vi "Command Handler.vi"(8 "error in (no error)":errorcluster, 11 "J1939 Main Configuration":T1={"Parameters"={"J1939 XNET Settings"={"XNET Database"="", "XNET Cluster"="", "CAN Port"="", "Baud rate [Bd]"=0, "Termination"=0, "Incoming Rate"=0, "Outcoming Rate"=1, "Write Decimation"=1}, "Incoming Single Point Configuraiton"={"ID"=[], "Conversion"=[], "Channel Array Positions"=[], "Frame Length"=[]}, "Outgoing Cyclic Configuraiton"={"ID"=[], "Conversion"=[], "Channel Array Positions"=[], "Frame Length"=[], "Transmit Propreties"=[]}, "J1939 Monitor Settings"={"J1939 Network Address"=0, "Name"=0}, "Simulated Addresses"=[], "Simulated Addresses LUT"=variant, "Name"=""}, "Name"="", "J1939 Cluster"={"Processed Incoming"=refnum, "Current Device Address"=0, "Processed Outgoing"=refnum, "Process Outgoing"=refnum, "Name"=0}, "References"={"BAM Buffer"=refnum, "CM Buffer"=refnum, "CM Gen"=refnum, "BAM Gen"=refnum, "Address Claims"=refnum, "RQST"=refnum}, "Frame In"="", "Frame Out"="", "Incoming Timeout"=0, "Outgoing Timeout"=0, "Process"=refnum, "Data Ref"=refnum, "Scale Ref"=refnum, "Incoming Direct Access"={"Offset"=0, "Length"=0}, "Outgoing Direct Access"={"Offset"=0, "Length"=0}, "Name and Address"="", "Simulated Addresses"=[], "Simulated Addresses LUT"=variant, "Outgoing"=refnum, "Incoming"=refnum, "Comm"=refnum} {"Simulated Addresses"."Simulated Addresses"."J1939 XNET Settings"."Name" format="%.0x"; "Simulated Addresses"."Simulated Addresses"."DM1 Data"."Data Reference" format="%.0x"; "Simulated Addresses"."Simulated Addresses"."DM1 Enable?"."Data Reference" format="%.0x"; "Simulated Addresses"."Simulated Addresses"."DM2 Data"."Data Reference" format="%.0x"; "Simulated Addresses"."Simulated Addresses"."DM2 Enable?"."Data Reference" format="%.0x"; "Parameters"."Simulated Addresses"."Simulated Addresses"."J1939 XNET Settings"."Name" format="%.0x"; "Parameters"."J1939 Monitor Settings"."Name" format="%.0x"; "Parameters"."Outgoing Cyclic Configuraiton"."Transmit Propreties"."Transmit Time" format="%#_p"; "Parameters"."J1939 XNET Settings"."Termination" items=["Off", "On"]}) -> (0 "error out":errorcluster)   [LabVIEW 2015, in "J1939 Addon Engine.lvlib"]
uses:
  J1939 Addon Engine.lvlib
  Types/Configuration Cluster.ctl
  <vilib>/NI/NIVS Inline Async API/_VS Inline Async API/Process/Process.lvclass
  <vilib>/NI/NIVS Addon Network Comm/Engine/VeriStand Comm.lvclass
  Types/Process Parameters.ctl
  Shared/Types/XNET Settings.ctl
  Types/Incoming Single Point Configuration.ctl
  Types/Outgoing Cyclic Configuration.ctl
  Shared/Types/XNET Frame Event Properties.ctl
  Shared/Types/Monitor Settings.ctl
  Types/Simulated Settings.ctl
  Shared/Types/Compiled Simulated Settings.ctl
  <vilib>/NI Veristand/Custom Device API/Block Data Reference.ctl
  <vilib>/NI Veristand/Custom Device API/Data Reference.ctl
  Types/DTC FIFOs.ctl
  J1939 Multi Packet Frame/Types/Setup Information Cluster.ctl
  <vilib>/xnet/xnet.llb/XNET Frame CAN.ctl
  <vilib>/xnet/xnet.llb/XNET Frame Type CAN.ctl
  Shared/J1939 Utilities/Types/CAN Outgoing Message Cluster.ctl
  J1939 Multi Packet Frame/Types/TP List References.ctl
  J1939 Multi Packet Frame/Types/BAM Buffer Connections List_Ref.ctl
  J1939 Multi Packet Frame/Types/TP Buffer Connection Cluster.ctl
  J1939 Multi Packet Frame/Types/Connection Mode Generation Connection Ref.ctl
  J1939 Multi Packet Frame/Types/Connection Mode Generation Connection Cluster.ctl
  J1939 Multi Packet Frame/Types/BAM Generation Connections List_Ref.ctl
  J1939 Multi Packet Frame/Types/BAM Generation Connection Cluster.ctl
  J1939 Multi Packet Frame/Types/Address Table Reference.ctl
  J1939 Multi Packet Frame/Types/RQST Lookup Table Reference.ctl
  Types/Data Lookup Table Reference.ctl
  Types/Datatable Lookup DVR.ctl
  Types/Conversion Lookup Table Reference.ctl
  <vilib>/NI/NIVS Inline Async API/_Data Access Engine/Access Type Classes/Read/Read.lvclass
  <vilib>/NI/NIVS Inline Async API/_Data Access Engine/Access Type Classes/Write/Write.lvclass
  <vilib>/NI/NIVS Addon Network Comm/Engine/VeriStand Comm.lvclass/VeriStand Comm.ctl
  Shared/Types/Request Message.ctl
  J1939 Multi Packet Frame/Types/Address Lookup Table Action.ctl
  <vilib>/NI/NIVS Inline Async API/_VS Inline Async API/Process/Process.lvclass/Process.ctl
  <vilib>/NI/NIVS Inline Async API/_VS Inline Async API/Error Handling Process/SubVIs/Error.ConvertArray.vi
  <vilib>/NI/AMC/Read Next Message.vi
  <vilib>/NI/Tools/Keyed Array/Index.vi
  Shared/J1939 Utilities/Common Messages.vi
  Shared/J1939 Utilities/SubVIs/Request.vi
  J1939 Multi Packet Frame/SubVIs/RQST Lookup Table Act.vi
  <vilib>/NI/AMC/Send Local Message.vi
  <vilib>/NI/AMC/Read Termination Message.vi
  <vilib>/NI/Tools/Keyed Array/Map String.vi
  Shared/J1939 Utilities/Common Conversions.vi
  Shared/J1939 Utilities/SubVIs/Convert J1939 ID to CAN Arb ID.vi
  <vilib>/NI/AMC/Create Single Message.vi
  <vilib>/NI/AMC/Update Message Routing Info.vi
  <vilib>/NI/Tools/String/Get Case Matching.vi
  <vilib>/NI/AMC/Send Message.vi
  J1939 Multi Packet Frame/SubVIs/Address Lookup Table.vi
  <vilib>/xnet/xnet.llb/XNET Read (State CAN Comm).vi
  J1939 Multi Packet Frame/SubVIs/RQST Lookup Table.vi
  <vilib>/NI/AMC/Globals.vi
  <vilib>/NI/NIVS Addon Network Comm/Shared/Comm Constants.vi
  Shared/J1939 Addon Shared.lvlib
  Shared/J1939 Utilities/J1939 Utilities.lvlib
  <vilib>/NI Veristand/Custom Device Tools/Custom Device Utility Library/Custom Device Utility Library.lvlib
  <vilib>/NI VeriStand/Custom Device API/Custom Device API.lvlib
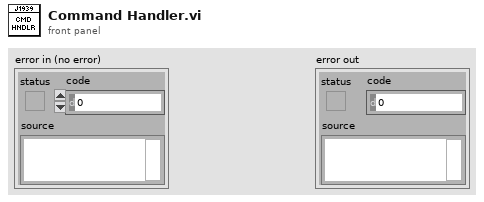
[diagram p1: front panel]
types:
  T1 = typedef "J1939 Addon Engine.lvlib/Configuration Cluster.ctl" = cluster{"Parameters":T2, "Name":string, "J1939 Cluster":T13, "References":T14, "Frame In":refnum<k21>, "Frame Out":refnum<k21>, "Incoming Timeout":u32, "Outgoing Timeout":u32, "Process":refnum<class "Process.lvclass">, "Data Ref":T20, "Scale Ref":T21, "Incoming Direct Access":cluster{"Offset":u32, "Length":u32}, "Outgoing Direct Access":cluster{"Offset":u32, "Length":u32}, "Name and Address":string, "Simulated Addresses":T8[], "Simulated Addresses LUT":variant, "Outgoing":refnum<data-value>, "Incoming":refnum<data-value>, "Comm":refnum<class "VeriStand Comm.lvclass">}
  T2 = typedef "J1939 Addon Engine.lvlib/Process Parameters.ctl" = cluster{"J1939 XNET Settings":T3, "Incoming Single Point Configuraiton":T4, "Outgoing Cyclic Configuraiton":T5, "J1939 Monitor Settings":T7, "Simulated Addresses":T8[], "Simulated Addresses LUT":variant, "Name":string}
  T3 = typedef "J1939 Addon Shared.lvlib/XNET Settings.ctl" = cluster{"XNET Database":refnum<k21>, "XNET Cluster":refnum<k21>, "CAN Port":string, "Baud rate [Bd]":u32, "Termination":u32, "Incoming Rate":u32, "Outcoming Rate":u32, "Write Decimation":u32}
  T4 = typedef "J1939 Addon Engine.lvlib/Incoming Single Point Configuration.ctl" = cluster{"ID":u32[], "Conversion":refnum<k21>[], "Channel Array Positions":cluster{"Offset":u32, "Length":u32}[], "Frame Length":u32[]}
  T5 = typedef "J1939 Addon Engine.lvlib/Outgoing Cyclic Configuration.ctl" = cluster{"ID":u32[], "Conversion":refnum<k21>[], "Channel Array Positions":cluster{"Offset":u32, "Length":u32}[], "Frame Length":u32[], "Transmit Propreties":T6[]}
  T6 = typedef "J1939 Addon Shared.lvlib/XNET Frame Event Properties.ctl" = cluster{"Transmit trigger":enum16{"Channel value change"}, "Enable software cyclic trigger":bool, "Transmit Time":dbl}
  T7 = typedef "J1939 Addon Shared.lvlib/Monitor Settings.ctl" = cluster{"J1939 Network Address":u8, "Name":u64}
  T8 = typedef "J1939 Addon Engine.lvlib/Simulated Settings.ctl" = cluster{"Simulated Addresses":T9, "FIFOs":T12}
  T9 = typedef "J1939 Addon Shared.lvlib/Compiled Simulated Settings.ctl" = cluster{"J1939 XNET Settings":T7, "DM1 Data":T10[], "DM1 Data":dbl[], "DM1 Enable?":T10[], "DM1 Enable?":dbl[], "DM2 Data":T10[], "DM2 Data":dbl[], "DM2 Enable?":T10[], "DM2 Enable?":dbl[]}
  T10 = typedef "Custom Device API.lvlib/Block Data Reference.ctl" = cluster{"Data Reference":T11, "Offset":u64, "Length":u64}
  T11 = typedef "Custom Device API.lvlib/Data Reference.ctl" = i32
  T12 = typedef "J1939 Addon Engine.lvlib/DTC FIFOs.ctl" = cluster{"DM1 Data":refnum<k33>, "DM1 Enable?":refnum<k33>, "DM2 Data":refnum<k33>, "DM2 Enable?":refnum<k33>, "DM1 Reset?":refnum<k33>, "DM2 Reset?":refnum<k33>}
  T13 = typedef "J1939 Addon Engine.lvlib/Setup Information Cluster.ctl" = cluster{"Processed Incoming":refnum<queue>, "Current Device Address":u8, "Processed Outgoing":refnum<queue>, "Process Outgoing":refnum<queue>, "Name":u64}
  T14 = typedef "J1939 Addon Engine.lvlib/TP List References.ctl" = cluster{"BAM Buffer":T15, "CM Buffer":T15, "CM Gen":T16, "BAM Gen":T17, "Address Claims":T18, "RQST":T19}
  T15 = typedef "J1939 Addon Engine.lvlib/BAM Buffer Connections List_Ref.ctl" = refnum<data-value>
  T16 = typedef "J1939 Addon Engine.lvlib/Connection Mode Generation Connection Ref.ctl" = refnum<data-value>
  T17 = typedef "J1939 Addon Engine.lvlib/BAM Generation Connections List_Ref.ctl" = refnum<data-value>
  T18 = typedef "J1939 Addon Engine.lvlib/Address Table Reference.ctl" = refnum<data-value>
  T19 = typedef "J1939 Addon Engine.lvlib/RQST Lookup Table Reference.ctl" = refnum<data-value>
  T20 = typedef "J1939 Addon Engine.lvlib/Data Lookup Table Reference.ctl" = refnum<data-value>
  T21 = typedef "J1939 Addon Engine.lvlib/Conversion Lookup Table Reference.ctl" = refnum<data-value>
  T22 = typedef "J1939 Addon Shared.lvlib/Request Message.ctl" = cluster{"PGN":u32, "DA":u8, "Ignore Response":bool}
  T23 = typedef "J1939 Addon Shared.lvlib/J1939 Utilities.lvlib/CAN Outgoing Message Cluster.ctl" = cluster{"Identifier":u32, "Data":u8[]}
  T24 = typedef "J1939 Addon Engine.lvlib/Address Lookup Table Action.ctl" = enum16{"Initialize", "Add", "Get", "Remove", "Get All"}
  T25 = typedef "NI VeriStand Addon Network Comm.lvlib/VeriStand Comm.lvclass/Response Information.ctl" = cluster{"response name":string, "responseQ":string}
  T26 = typedef "XNET Frame CAN.ctl" = cluster{"timestamp":timestamp, "payload":u8[], "identifier":u32, "type":T27, "extended?":bool, "echo?":bool}
  T27 = typedef "XNET Frame Type CAN.ctl" = u8
  T28 = typedef "XNET CAN Comm.ctl" = cluster{"fault code":i32, "fault?":bool, "communication state":T29, "last error":T30, "receive error counter":u8, "transmit error counter":u8, "transceiver error?":bool, "sleep?":bool}
  T29 = typedef "XNET CAN Comm State.ctl" = u8
  T30 = typedef "XNET CAN Last Err.ctl" = u8
  T31 = typedef "J1939 Addon Shared.lvlib/Address Lookup Table Data.ctl" = cluster{"Name":u8[], "Address":u8}
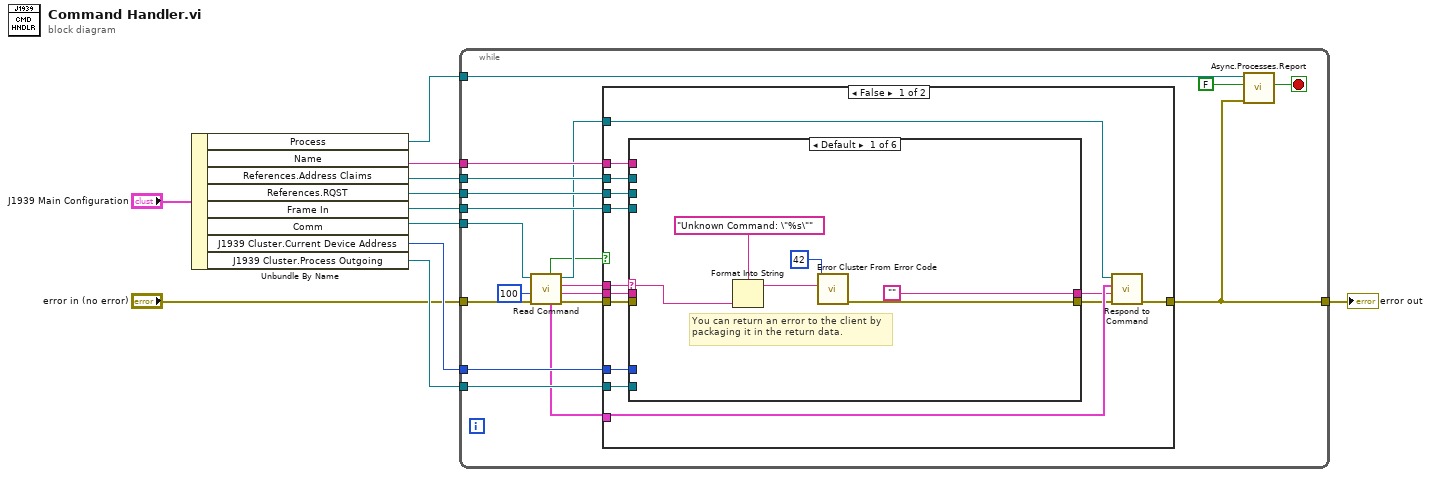
[diagram p0: block diagram]
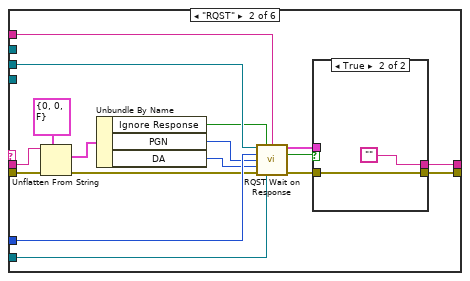
[diagram p2: hidden frame]
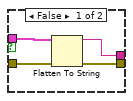
[diagram p3: hidden frame]
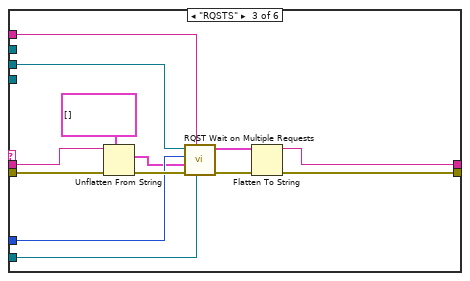
[diagram p4: hidden frame]
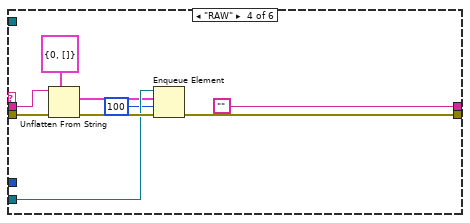
[diagram p5: hidden frame]
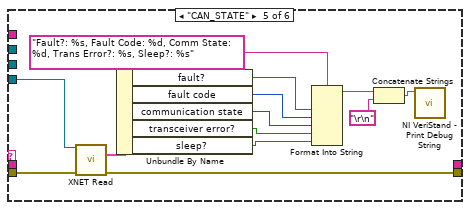
[diagram p6: hidden frame]
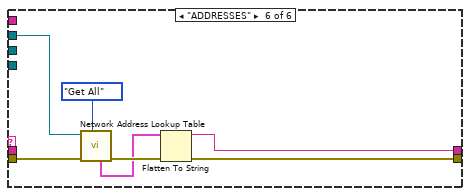
[diagram p7: hidden frame]
diagram:
  n1 = Unbundle By Name("J1939 Main Configuration") -> ("Process"=w11:refnum<class "Process.lvclass">, "Name"=w10:string, "References.Address Claims"=w9:T18, "References.RQST"=w8:T19, "Frame In"=w7:refnum<k21>, "Comm"=w6:refnum<class "VeriStand Comm.lvclass">, "J1939 Cluster.Current Device Address"=w5:u8, "J1939 Cluster.Process Outgoing"=w4:refnum<queue>)
  n2 = while {
    tunnel: "error in (no error)" -> [w27]
    tunnel: [w19] -> w1
    tunnel: w11 -> [w29]
    tunnel: w6 -> [w26]
    tunnel: w10 -> [w25]
    tunnel: w7 -> [w24]
    tunnel: w4 -> [w23]
    tunnel: w5 -> [w22]
    tunnel: w8 -> [w21]
    tunnel: w9 -> [w20]
    stop <- w30 stop-if-true
    n3 = call <vilib>:"Read Command.vi"("error in (no error)"=w27, "timeout (100 ms)"=100, "VeriStand Comm in"=w26) -> ("error out"=w17:errorcluster, "message value"=w15:string, "message name"=w16:string, "VeriStand Comm out"=w13:refnum<class "VeriStand Comm.lvclass">, "ResponseInfo"=w14:T25, "timed out?"=w12:bool)  [unwired: 3 in]
    n4 = case shown="False" w12 {
      tunnel: w25 -> [w44 _]
      tunnel: w24 -> [w43 _]
      tunnel: w23 -> [w42 _]
      tunnel: w22 -> [w41 _]
      tunnel: w21 -> [w40 _]
      tunnel: w20 -> [w39 _]
      tunnel: [w38 w116] -> w19
      tunnel: w17 -> [w37 w116]
      tunnel: w16 -> [w36 _]
      tunnel: w15 -> [w35 _]
      tunnel: w14 -> [w34 _]
      tunnel: w13 -> [w33 _]
      frame False {
        n5 = case shown="Default" w36 {
          selector: w36 -> [w46 _ _ _ _ _]
          tunnel: w35 -> [_ w54 w83 w94 _ _]
          tunnel: [w47 w66 w86 w88 w106 w109] -> w31
          tunnel: ["" ("data string") w63 w85 "" _ w110] -> w32
          tunnel: w42 -> [_ w61 w80 w91 _ _]
          tunnel: w37 -> [_ w60 w84 w95 w108 w114]
          tunnel: w40 -> [_ w53 w78 _ _ _]
          tunnel: w41 -> [_ w67 w77 _ _ _]
          tunnel: w39 -> [_ _ _ _ _ w113]
          tunnel: w44 -> [_ w51 w74 _ _ _]
          tunnel: w43 -> [_ _ _ _ w107 _]
          frame Default {
            # "You can return an error to the client by packaging it in the return data."
            n6 = Format Into String(format string="Unknown Command: \"%s\"", w46) -> (resulting string=w48:string)  [unwired: 2 in, 1 out]
            n7 = call <vilib>:"Error Cluster From Error Code.vi"("error message (\"\")"=w48, "error code (0)"=42) -> ("error out"=w47:errorcluster)  [unwired: 7 in]
          }
          frame "RQST" {
            n8 = Unflatten From String(type=T22 {"PGN"=0, "DA"=0, "Ignore Response"=FALSE} ("Cluster"), binary string=w54, error in (no error)=w60) -> (value=w57:T22, error out=w59:errorcluster)  [unwired: 2 in, 1 out]
            n9 = Unbundle By Name(w57) -> ("Ignore Response"=w52:bool, "PGN"=w56:u32, "DA"=w55:u8)
            n10 = call "RQST Wait on Response.vi"("ref in"=w53, "Ignore Response"=w52, "Name"=w51, "Source Address"=w67, "PGN"=w56, "DA"=w55, "error in (no error)"=w59, "Processed Outgoing"=w61) -> ("element"=w62:T26, "timed out?"=w64:bool, "error out"=w65:errorcluster)  [unwired: 4 in, 1 out]
            n11 = case shown="True" w64 {
              tunnel: [w69 w73] -> w66
              tunnel: w65 -> [w70 w73]
              tunnel: [w68 ""] -> w63
              tunnel: w62 -> [w71 _]
              frame False {
                n12 = Flatten To String(anything=w71, error in (no error)=w70) -> (data string=w68:string, error out=w69:errorcluster)  [unwired: 2 in, 1 out]
              }
              frame True {
              }
            }
          }
          frame "RQSTS" {
            n13 = Unflatten From String(type=T22[] [], binary string=w83, error in (no error)=w84) -> (value=w76:T22[], error out=w81:errorcluster)  [unwired: 2 in, 1 out]
            n14 = call "RQST Wait on Multiple Requests.vi"("Processed Outgoing"=w80, "Name"=w74, "error in (no error)"=w81, "value"=w76, "Source Address"=w77, "ref in"=w78) -> ("error out"=w79:errorcluster, "Elements"=w75:T26[])  [unwired: 2 in, 2 out]
            n15 = Flatten To String(anything=w75, error in (no error)=w79) -> (data string=w85:string, error out=w86:errorcluster)  [unwired: 2 in, 1 out]
          }
          frame "RAW" {
            n16 = Unflatten From String(type=T23 {"Identifier"=0, "Data"=[]} ("Data to Send"), binary string=w94, error in (no error)=w95) -> (value=w90:T23, error out=w92:errorcluster)  [unwired: 2 in, 1 out]
            n17 = Enqueue Element(queue=w91, element=w90, timeout in ms (-1)=100, error in (no error)=w92) -> (error out=w88:errorcluster)  [unwired: 2 out]
          }
          frame "CAN_STATE" {
            n18 = call-poly <vilib>:"XNET Read.vi"("session in"=w107, "error in (no error)"=w108) -> ("CAN comm"=w105:T28, "error out"=w106:errorcluster)  [unwired: 11 in, 1 out]
            n19 = Unbundle By Name(w105) -> ("fault?"=w104:bool, "fault code"=w103:i32, "communication state"=w102:T29, "transceiver error?"=w101:bool, "sleep?"=w100:bool)
            n20 = Format Into String(format string="Fault?: %s, Fault Code: %d, Comm State: %d, Trans Error?: %s, Sleep?: %s", w104, w103, w102, w101, w100) -> (resulting string=w99:string)  [unwired: 2 in, 1 out]
            n21 = Concatenate Strings(w99, "\r\n") -> (w97:string)
            n22 = call <vilib>:"NI VeriStand - Print Debug String.vi"("Message"=w97) -> ()  [unwired: 10 in, 1 out]
          }
          frame "ADDRESSES" {
            n23 = call "Network Address Lookup Table.vi"("Action"=Address_Lookup_Table_Action."Get All", "error in (no error)"=w114, "Address LUT"=w113) -> ("error out"=w112:errorcluster, "All Data"=w111:T31[])  [unwired: 4 in, 3 out]
            n24 = Flatten To String(anything=w111, error in (no error)=w112) -> (data string=w110:string, error out=w109:errorcluster)  [unwired: 2 in, 1 out]
          }
        }
        n25 = call <vilib>:"Respond to Command.vi"("error in (no error)"=w31, "message value"=w32, "ResponseInfo"=w34, "VeriStand Comm in"=w33) -> ("error out"=w38:errorcluster)  [unwired: 5 in, 2 out]
      }
      frame True {
      }
    }
    n26 = call <vilib>:"Async.Processes.Report.vi"("Error"=w19, "Stop Async on Error?"=FALSE ("Stop on Error?"), "Process in"=w29) -> ("Stop"=w30:bool)  [unwired: 7 in, 1 out]
  }
  "error out" <- w1
